vi "CH3_Tx.vi"() -> ()   [LabVIEW 2018]
uses:
  Stream/Stream.lvclass
  RxTx/RxTx.lvclass
panel:
  in  "RxTx.lvclass":refnum<class "RxTx.lvclass">
  in  "Stream.lvclass":refnum<class "Stream.lvclass">
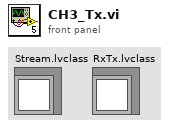
[diagram p1: front panel]
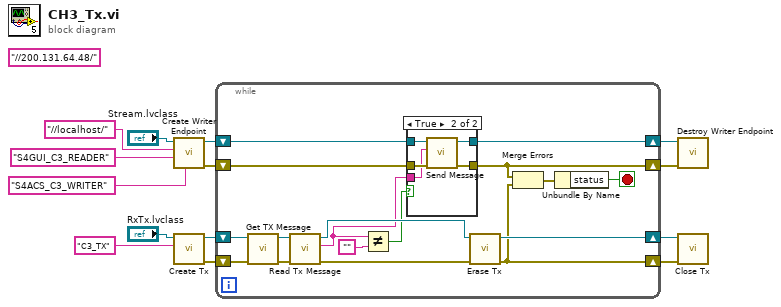
[diagram p0: block diagram]
diagram:
  (unwired) "//200.131.64.48/" ("Reader Name")
  n1 = call "Create Writer Endpoint.vi"("writer name"="S4ACS_C3_WRITER" ("reader name"), "reader name"="S4GUI_C3_READER", "IP"="//localhost/" ("Reader Name"), "Stream in"="Stream.lvclass") -> ("error out"=w6:errorcluster, "Stream out"=w8:refnum<class "Stream.lvclass">)  [unwired: 6 in]
  n2 = call "Create Tx.vi"("Writer Name"="C3_TX" ("Reader Name"), "RxTx in"="RxTx.lvclass") -> ("error out"=w12:errorcluster, "RxTx out"=w13:refnum<class "RxTx.lvclass">)  [unwired: 8 in]
  n3 = while {
    shift-right: [w23] -> w4
    shift-left: w6 -> [w25]
    shift-right: [w24] -> w14
    shift-left: w8 -> [w26]
    shift-right: [w18] -> w9
    shift-left: w12 -> [w27]
    shift-right: [w20] -> w10
    shift-left: w13 -> [w28]
    stop <- w15 stop-if-true
    n4 = call "Get TX Message.vi"("error in (no error)"=w27, "RxTx in"=w28) -> ("error out"=w30:errorcluster, "RxTx out"=w29:refnum<class "RxTx.lvclass">)  [unwired: 8 in]
    n5 = call "Read Tx Message.vi"("error in (no error)"=w30, "RxTx in"=w29) -> ("error out"=w19:errorcluster, "Tx Message"=w17:string, "RxTx out"=w21:refnum<class "RxTx.lvclass">)  [unwired: 7 in]
    n6 = Not Equal?(x=w17, y="") -> (x != y?=w16:bool)
    n7 = case shown="True" w16 {
      tunnel: w26 -> [w33 w38]
      tunnel: w25 -> [w32 w37]
      tunnel: [w33 w36] -> w24
      tunnel: w17 -> [_ w35]
      tunnel: [w32 w34] -> w23
      frame False {
      }
      frame True {
        n8 = call "Send Message.vi"("error in (no error)"=w37, "Message"=w35, "Stream in"=w38) -> ("error out"=w34:errorcluster, "Stream out"=w36:refnum<class "Stream.lvclass">)  [unwired: 7 in]
      }
    }
    n9 = call "Erase Tx.vi"("error in (no error)"=w19, "RxTx in"=w21) -> ("error out"=w18:errorcluster, "RxTx out"=w20:refnum<class "RxTx.lvclass">)  [unwired: 8 in]
    n10 = Merge Errors(w23, w18) -> (w31:errorcluster)
    n11 = Unbundle By Name(w31) -> ("status"=w15:bool)
  }
  n12 = call "Destroy Writer Endpoint.vi"("error in (no error)"=w4, "Stream in"=w14) -> ()  [unwired: 8 in, 2 out]
  n13 = call "Close Tx.vi"("error in (no error)"=w9, "RxTx in"=w10) -> ()  [unwired: 8 in, 2 out]
